vi "Refresh Listbox Data to Sysdef Data.vi"(8 "error in":errorcluster, 10 "Refresh Listbox":T4) -> (0 "error out":errorcluster, 2 "Refresh Sysdef":T1[](array[typedef]))   [LabVIEW 2020, in "Communication Bus Template System Explorer.lvlib" / "Implementation.lvlib"]
uses:
  Implementation.lvlib
  Types/Signal.ctl
  Types/Frame.ctl
  Types/Refresh For Sysdef.ctl
  Types/Refresh Listbox.ctl
  Types/Refresh Symbols.ctl
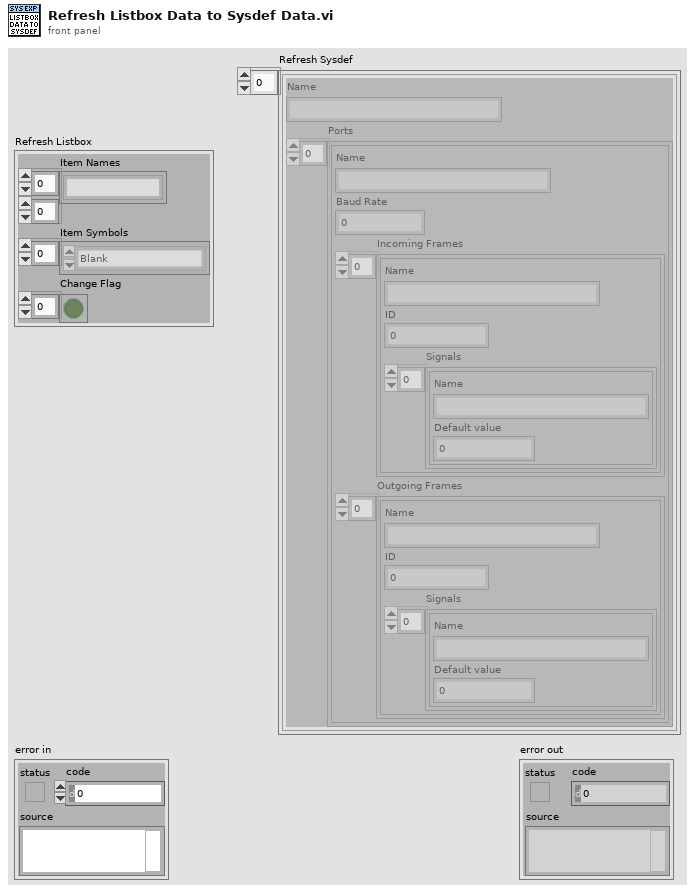
[diagram p1: front panel]
types:
  T1 = typedef "Communication Bus Template System Explorer.lvlib/Implementation.lvlib/Refresh For Sysdef.ctl" = cluster{"Name":string, "Ports":cluster{"Name":string, "Baud Rate":u64, "Incoming Frames":T2[], "Outgoing Frames":T2[]}[]}
  T2 = typedef "Communication Bus Template System Explorer.lvlib/Implementation.lvlib/Frame.ctl" = cluster{"Name":string, "ID":u32, "Signals":T3[]}
  T3 = typedef "Communication Bus Template System Explorer.lvlib/Implementation.lvlib/Signal.ctl" = cluster{"Name":string, "Default value":dbl}
  T4 = typedef "Communication Bus Template System Explorer.lvlib/Implementation.lvlib/Refresh Listbox.ctl" = cluster{"Item Names":string[][], "Item Symbols":T5[], "Change Flag":bool[]}
  T5 = typedef "Communication Bus Template System Explorer.lvlib/Implementation.lvlib/Refresh Symbols.ctl" = enum16{"Blank", "Port", "Incoming", "Outgoing", "Frame", "Signal", "Cluster", "Baud Rate"}
  T6 = cluster{"Name":string, "Ports":cluster{"Name":string, "Baud Rate":u64, "Incoming Frames":T2[], "Outgoing Frames":T2[]}[]}
  T7 = cluster{"Name":string, "Baud Rate":u64, "Incoming Frames":T2[], "Outgoing Frames":T2[]}
  T8 = cluster{"Name":string, "Baud Rate":u64, "Incoming Frames":T2[], "Outgoing Frames":T2[]}[]
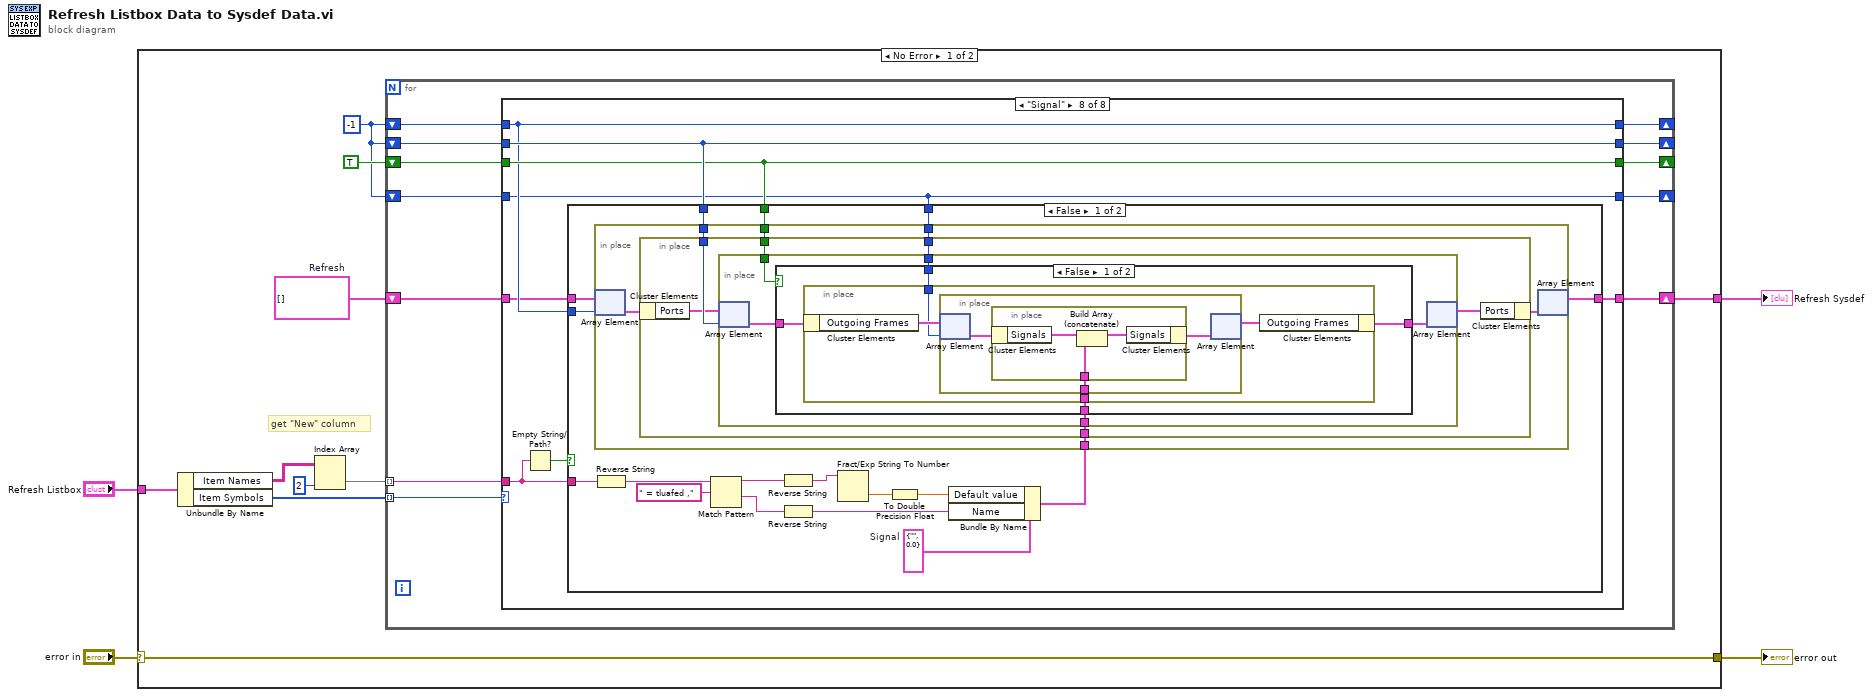
[diagram p0: block diagram]
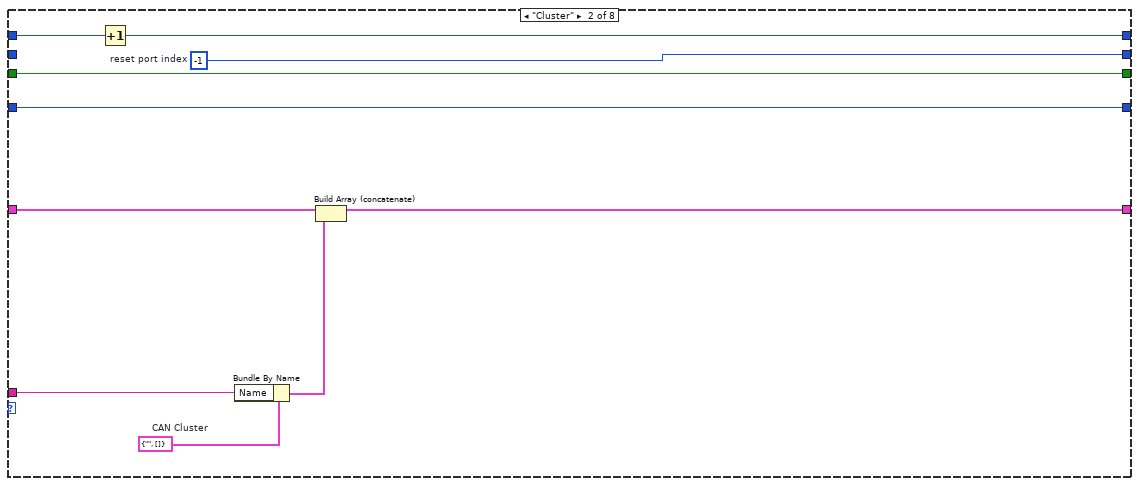
[diagram p3: hidden frame]
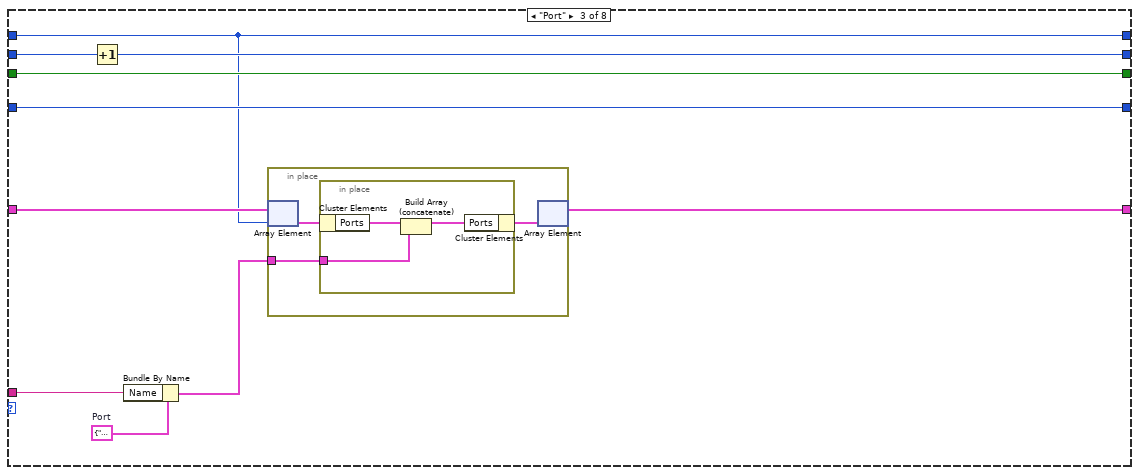
[diagram p4: hidden frame]
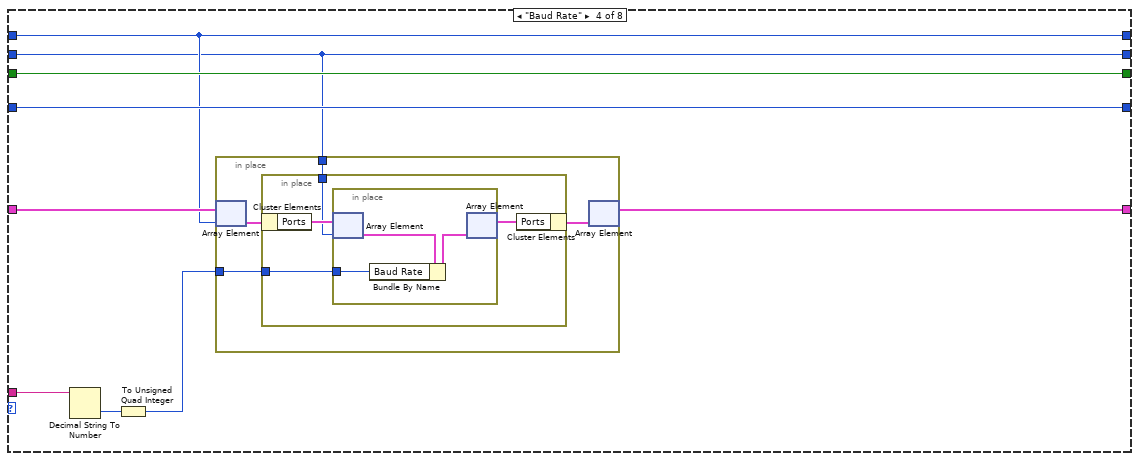
[diagram p5: hidden frame]
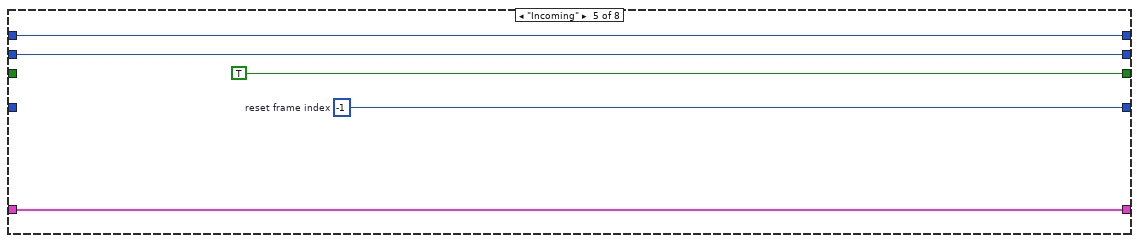
[diagram p6: hidden frame]
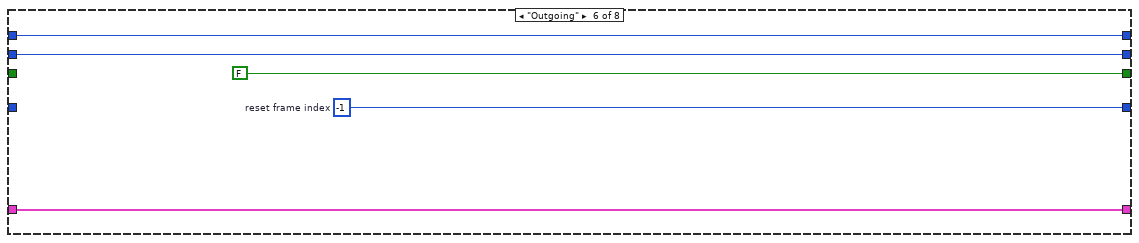
[diagram p7: hidden frame]
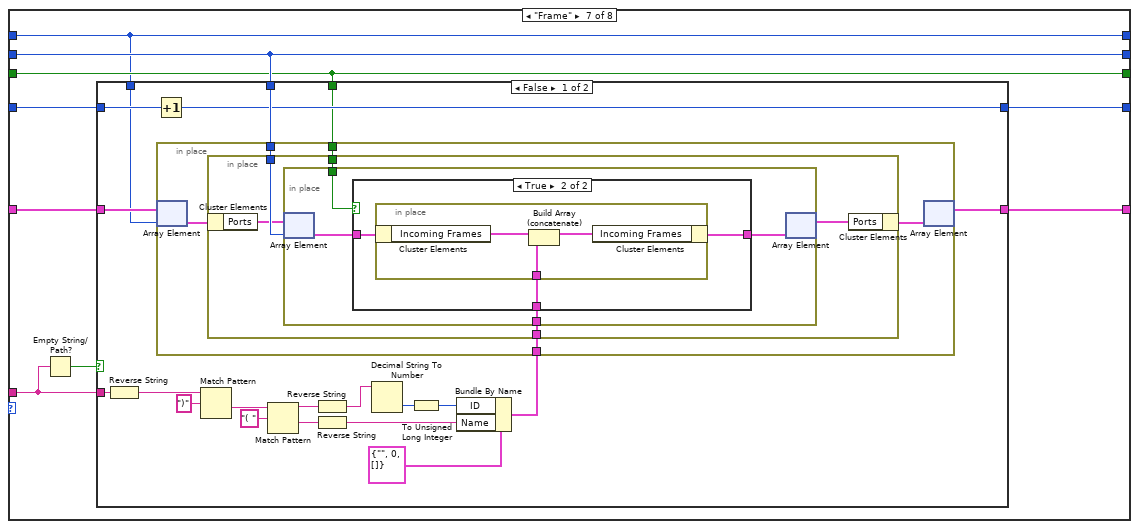
[diagram p8: hidden frame]
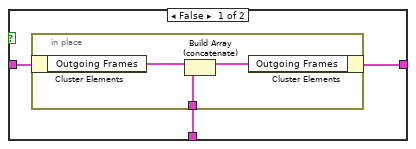
[diagram p9: hidden frame]
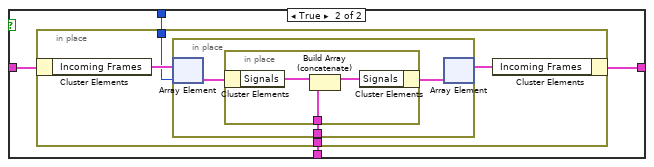
[diagram p11: hidden frame]
diagram:
  n1 = case shown="No Error" "error in" {
    selector: "error in" -> [w5 w216]
    tunnel: "Refresh Listbox" -> [w14 _]
    tunnel: [w6 _] -> w3
    tunnel: [w5 w216] -> w1
    frame No Error {
      w7 = T1[] []  # Refresh
      w8 = -1
      # "get \"New\" column"
      n2 = Unbundle By Name(w14) -> ("Item Names"=w10:string[][], "Item Symbols"=w13:T5[])
      n3 = Index Array(array=w10, index (col)=2 ("disabled index (col)")) -> (element=w11:string[])  [unwired: 1 in]
      n4 = for {
        tunnel: w13 -> [w26] mode=indexing
        tunnel: w11 -> [w25] mode=indexing
        shift-right: [w23] -> w6
        shift-left: w7 -> [w24]
        shift-right: [w21] -> _
        shift-left: w8 -> [w22]
        shift-right: [w19] -> _
        shift-left: w8 -> [w20]
        shift-right: [w17] -> _
        shift-left: TRUE -> [w18]
        shift-right: [w15] -> _
        shift-left: w8 -> [w16]
        n5 = case shown="\"Signal\"" w26 {
          tunnel: w25 -> [_ w40 w50 w65 _ _ w89 w146]
          tunnel: w24 -> [w28 w41 w49 w66 w79 w84 w92 w149]
          tunnel: [w28 w38 w44 w61 w79 w84 w90 w148] -> w23
          tunnel: w22 -> [w31 w37 w43 w62 w82 w87 w91 w150]
          tunnel: [w31 w36 w43 w62 w82 w87 w91 w150] -> w21
          tunnel: w20 -> [w30 _ w48 w60 w81 w86 w96 w152]
          tunnel: [w30 w33 w47 w60 w81 w86 w96 w152] -> w19
          tunnel: w18 -> [w29 w35 w46 w64 _ _ w93 w151]
          tunnel: [w29 w35 w46 w64 TRUE FALSE w93 w151] -> w17
          tunnel: w16 -> [w27 w34 w45 w63 _ _ w95 w147]
          tunnel: [w27 w34 w45 w63 w78 w83 w94 w147] -> w15
          frame "Blank", Default {
          }
          frame "Cluster" {
            w32 = T6 {"Name"="", "Ports"=[]}  # CAN Cluster
            w33 = -1  # reset port index
            n6 = Increment(x=w37) -> (x+1=w36:i32)
            n7 = Bundle By Name(cluster=w32, "Name"=w40) -> (w39:T6)
            n8 = Build Array (concatenate)(w41, w39) -> (w38:T1[])
          }
          frame "Port" {
            w51 = T7 {"Name"="", "Baud Rate"=0, "Incoming Frames"=[], "Outgoing Frames"=[]}  # Port
            n9 = Increment(x=w48) -> (x+1=w47:i32)
            n10 = Bundle By Name(cluster=w51, "Name"=w50) -> (w42:T7)
            n11 = in-place {
              in-place-border: w42 -> [w53]
              n12 = in-place-array #1(w49, w43) -> (w54:T1)
              n13 = in-place {
                in-place-border: w53 -> [w56]
                n14 = in-place-cluster #2(w54) -> ("Ports"=w57:T8)
                n15 = Build Array (concatenate)(w57, w56) -> (w55:T8)
                n16 = in-place-cluster #2("Ports"=w55) -> (w52:T1)
              }
              n17 = in-place-array #1(w52) -> (w44:T1[])  [unwired: 1 out]
            }
          }
          frame "Baud Rate" {
            n18 = Decimal String To Number(string=w65) -> (number=w59:i32)  [unwired: 2 in, 1 out]
            n19 = To Unsigned Quad Integer(1:w59) -> (0:w58:u64)
            n20 = in-place {
              in-place-border: w60 -> [w69]
              in-place-border: w58 -> [w67]
              n21 = in-place-array #3(w66, w62) -> (w70:T1)
              n22 = in-place {
                in-place-border: w69 -> [w73]
                in-place-border: w67 -> [w71]
                n23 = in-place-cluster #4(w70) -> ("Ports"=w74:T8)
                n24 = in-place {
                  in-place-border: w71 -> [w75]
                  n25 = in-place-array #5(w74, w73) -> (w77:T7)
                  n26 = Bundle By Name(cluster=w77, "Baud Rate"=w75) -> (w76:T7)
                  n27 = in-place-array #5(w76) -> (w72:T8)  [unwired: 1 out]
                }
                n28 = in-place-cluster #4("Ports"=w72) -> (w68:T1)
              }
              n29 = in-place-array #3(w68) -> (w61:T1[])  [unwired: 1 out]
            }
          }
          frame "Incoming" {
            w78 = -1  # reset frame index
          }
          frame "Outgoing" {
            w83 = -1  # reset frame index
          }
          frame "Frame" {
            n30 = Empty String/Path?(string/path=w89) -> (empty?=w88:bool)
            n31 = case shown="False" w88 {
              tunnel: w89 -> [w116 _]
              tunnel: w96 -> [w103 _]
              tunnel: w95 -> [w102 w144]
              tunnel: [w101 w144] -> w94
              tunnel: w93 -> [w100 _]
              tunnel: w92 -> [w99 w143]
              tunnel: w91 -> [w98 _]
              tunnel: [w97 w143] -> w90
              frame False {
                n32 = Reverse String(1:w116) -> (0:w115:string)
                n33 = Increment(x=w102) -> (x+1=w101:i32)
                n34 = Match Pattern(string=w115, regular expression=")") -> (after substring=w112:string)  [unwired: 1 in, 3 out]
                n35 = Match Pattern(string=w112, regular expression="( ") -> (before substring=w111:string, after substring=w110:string)  [unwired: 1 in, 2 out]
                n36 = Reverse String(1:w111) -> (0:w107:string)
                n37 = Reverse String(1:w110) -> (0:w109:string)
                n38 = Decimal String To Number(string=w107) -> (number=w106:i32)  [unwired: 2 in, 1 out]
                n39 = To Unsigned Long Integer(number=w106) -> (unsigned 32bit integer=w105:u32)
                n40 = Bundle By Name(cluster=T2 {"Name"="", "ID"=0, "Signals"=[]} ("Frame"), "ID"=w105, "Name"=w109) -> (w104:T2)
                n41 = in-place {
                  in-place-border: w104 -> [w121]
                  in-place-border: w103 -> [w120]
                  in-place-border: w100 -> [w119]
                  n42 = in-place-array #6(w99, w98) -> (w118:T1)
                  n43 = in-place {
                    in-place-border: w121 -> [w126]
                    in-place-border: w120 -> [w124]
                    in-place-border: w119 -> [w125]
                    n44 = in-place-cluster #7(w118) -> ("Ports"=w123:T8)
                    n45 = in-place {
                      in-place-border: w126 -> [w130]
                      in-place-border: w125 -> [w129]
                      n46 = in-place-array #8(w123, w124) -> (w128:T7)
                      n47 = case shown="True" w129 {
                        tunnel: w130 -> [w133 w139]
                        tunnel: w128 -> [w132 w138]
                        tunnel: [w131 w137] -> w127
                        frame False {
                          n48 = in-place {
                            in-place-border: w133 -> [w136]
                            n49 = in-place-cluster #9(w132) -> ("Outgoing Frames"=w135:T2[])
                            n50 = Build Array (concatenate)(w135, w136) -> (w134:T2[])
                            n51 = in-place-cluster #9("Outgoing Frames"=w134) -> (w131:T7)
                          }
                        }
                        frame True {
                          n52 = in-place {
                            in-place-border: w139 -> [w142]
                            n53 = in-place-cluster #10(w138) -> ("Incoming Frames"=w141:T2[])
                            n54 = Build Array (concatenate)(w141, w142) -> (w140:T2[])
                            n55 = in-place-cluster #10("Incoming Frames"=w140) -> (w137:T7)
                          }
                        }
                      }
                      n56 = in-place-array #8(w127) -> (w122:T8)  [unwired: 1 out]
                    }
                    n57 = in-place-cluster #7("Ports"=w122) -> (w117:T1)
                  }
                  n58 = in-place-array #6(w117) -> (w97:T1[])  [unwired: 1 out]
                }
              }
              frame True {
              }
            }
          }
          frame "Signal" {
            n59 = Empty String/Path?(string/path=w146) -> (empty?=w145:bool)
            n60 = case shown="False" w145 {
              tunnel: w146 -> [w169 _]
              tunnel: w152 -> [w162 _]
              tunnel: w151 -> [w157 _]
              tunnel: w150 -> [w156 _]
              tunnel: w149 -> [w155 w215]
              tunnel: [w154 w215] -> w148
              tunnel: w147 -> [w153 _]
              frame False {
                w159 = T3 {"Name"="", "Default value"=0.0}  # Signal
                n61 = Reverse String(1:w169) -> (0:w168:string)
                n62 = Match Pattern(string=w168, regular expression=" = tluafed ,") -> (before substring=w161:string, after substring=w160:string)  [unwired: 1 in, 2 out]
                n63 = Reverse String(1:w161) -> (0:w165:string)
                n64 = Reverse String(1:w160) -> (0:w166:string)
                n65 = Fract/Exp String To Number(string=w165) -> (number=w164:dbl)  [unwired: 3 in, 1 out]
                n66 = To Double Precision Float(number=w164) -> (double precision float=w163:dbl)
                n67 = Bundle By Name(cluster=w159, "Default value"=w163, "Name"=w166) -> (w158:T3)
                n68 = in-place {
                  in-place-border: w162 -> [w175]
                  in-place-border: w158 -> [w174]
                  in-place-border: w157 -> [w173]
                  in-place-border: w153 -> [w171]
                  n69 = in-place-array #11(w155, w156) -> (w172:T1)
                  n70 = in-place {
                    in-place-border: w175 -> [w179]
                    in-place-border: w174 -> [w181]
                    in-place-border: w173 -> [w180]
                    in-place-border: w171 -> [w177]
                    n71 = in-place-cluster #12(w172) -> ("Ports"=w178:T8)
                    n72 = in-place {
                      in-place-border: w181 -> [w186]
                      in-place-border: w180 -> [w185]
                      in-place-border: w177 -> [w182]
                      n73 = in-place-array #13(w178, w179) -> (w184:T7)
                      n74 = case shown="False" w185 {
                        tunnel: w184 -> [w189 w203]
                        tunnel: w186 -> [w190 w204]
                        tunnel: [w188 w202] -> w183
                        tunnel: w182 -> [w187 w201]
                        frame False {
                          n75 = in-place {
                            in-place-border: w190 -> [w194]
                            in-place-border: w187 -> [w192]
                            n76 = in-place-cluster #14(w189) -> ("Outgoing Frames"=w193:T2[])
                            n77 = in-place {
                              in-place-border: w194 -> [w197]
                              n78 = in-place-array #15(w193, w192) -> (w196:T2)
                              n79 = in-place {
                                in-place-border: w197 -> [w200]
                                n80 = in-place-cluster #16(w196) -> ("Signals"=w199:T3[])
                                n81 = Build Array (concatenate)(w199, w200) -> (w198:T3[])
                                n82 = in-place-cluster #16("Signals"=w198) -> (w195:T2)
                              }
                              n83 = in-place-array #15(w195) -> (w191:T2[])  [unwired: 1 out]
                            }
                            n84 = in-place-cluster #14("Outgoing Frames"=w191) -> (w188:T7)
                          }
                        }
                        frame True {
                          n85 = in-place {
                            in-place-border: w204 -> [w208]
                            in-place-border: w201 -> [w206]
                            n86 = in-place-cluster #17(w203) -> ("Incoming Frames"=w207:T2[])
                            n87 = in-place {
                              in-place-border: w208 -> [w211]
                              n88 = in-place-array #18(w207, w206) -> (w210:T2)
                              n89 = in-place {
                                in-place-border: w211 -> [w214]
                                n90 = in-place-cluster #19(w210) -> ("Signals"=w213:T3[])
                                n91 = Build Array (concatenate)(w213, w214) -> (w212:T3[])
                                n92 = in-place-cluster #19("Signals"=w212) -> (w209:T2)
                              }
                              n93 = in-place-array #18(w209) -> (w205:T2[])  [unwired: 1 out]
                            }
                            n94 = in-place-cluster #17("Incoming Frames"=w205) -> (w202:T7)
                          }
                        }
                      }
                      n95 = in-place-array #13(w183) -> (w176:T8)  [unwired: 1 out]
                    }
                    n96 = in-place-cluster #12("Ports"=w176) -> (w170:T1)
                  }
                  n97 = in-place-array #11(w170) -> (w154:T1[])  [unwired: 1 out]
                }
              }
              frame True {
              }
            }
          }
        }
      }
    }
    frame Error {
    }
  }
  "error out" <- w1
  "Refresh Sysdef" <- w3
